vi "asap_signals.vi"() -> (1 "ASAP signals":sgl[][](array[numeric]), 2 "Num lights":i32)   [LabVIEW 2013]
panel:
  # "Return number of lights and current ASAP signals, as pushed out by asap_monitor.vi.  See also averaged_asap_signals.vi."
  # "Lights"
  # "Channel 0"
  # "Channel 7"
  # "X"
  # "Y"
  # "Z"
  # "Match error"
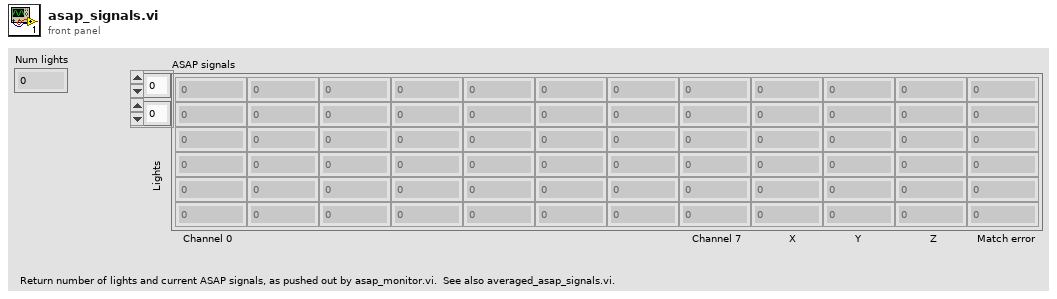
[diagram p1: front panel]
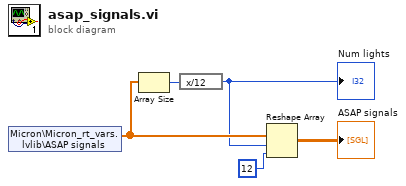
[diagram p0: block diagram]
diagram:
  n1 = shared-variable "Micron\\Micron_rt_vars.lvlib\\ASAP signals"() -> (w5:sgl[])  [unwired: 1 in, 1 out]
  n2 = Array Size(array=w5) -> (size(s)=w4:i32)
  n3 = expression code="x/12"(w4) -> (w2:i32)
  "Num lights" <- w2
  n4 = Reshape Array(w5, w2, 12 ("dimension size")) -> (→"ASAP signals":sgl[][])
